vi "Measure-Scope.vi"(0 "VISA resource name":refnum<visa-resource-name>, 1 "Avg Num Samples":dbl, 3 "Boolean":bool, 5 "Channel1 (0:Channel1)":u16(ring) items=["Channel1", "Channel2", "Channel3", "Channel4", "Math1", "Math2", "Math3", "Math3", "Reference1", "Reference2", "Reference3", "Reference4"], 9 "Gate Index":i32, 11 "Gate Length":i32=1000, 12 "error in (no error)":errorcluster) -> (4 "Full Waveform":waveform(dbl)(graph)={"t0"=timestamp(1.815305999999491e-07 s since 1904-01-01), "dt"=5e-07, "Y"=array[10000 elements]}, 6 "Gate":dbl[](graph), 8 "Signal Duration (ns)":dbl, 10 "Signal Arrival (ns)":dbl, 14 "Sum of Intensity (V)":dbl, 15 "Wait Time (ms)":dbl)   [LabVIEW 2018]
uses:
  <instrlib>/Tektronix 7000 Series/Public/Data/Read Waveform Measurement (More).vi
  <instrlib>/Tektronix 7000 Series/Public/Data/Read (Single Waveform).vi
  <instrlib>/Tektronix 7000 Series/Tektronix 7000 Series.lvlib
panel:
  out "Area (V*s)":dbl
  in  "Function(0:Amplitude)":u16(ring) items=["Area", "Burst Width", "Cyc Area", "Phase"]
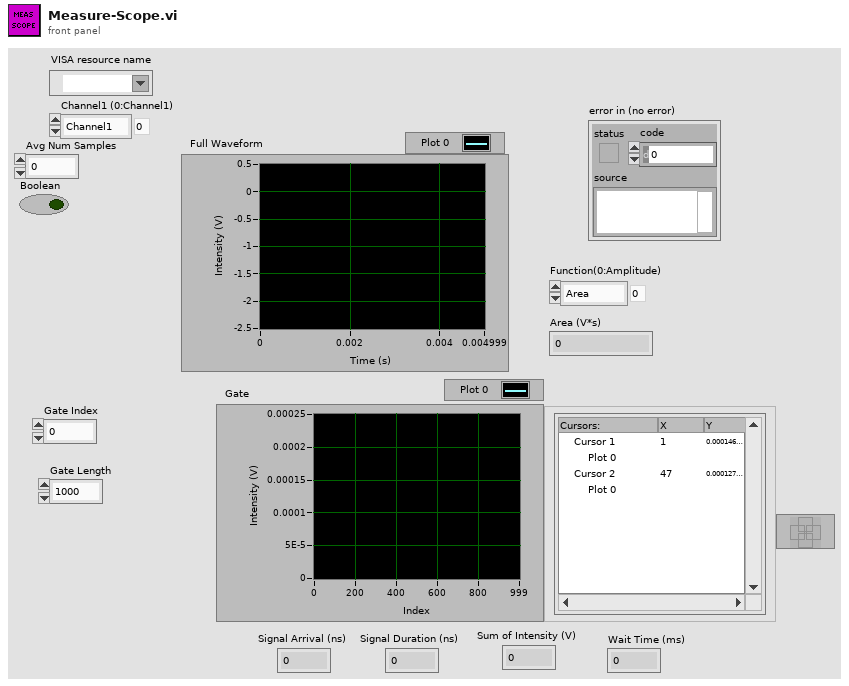
[diagram p1: front panel]
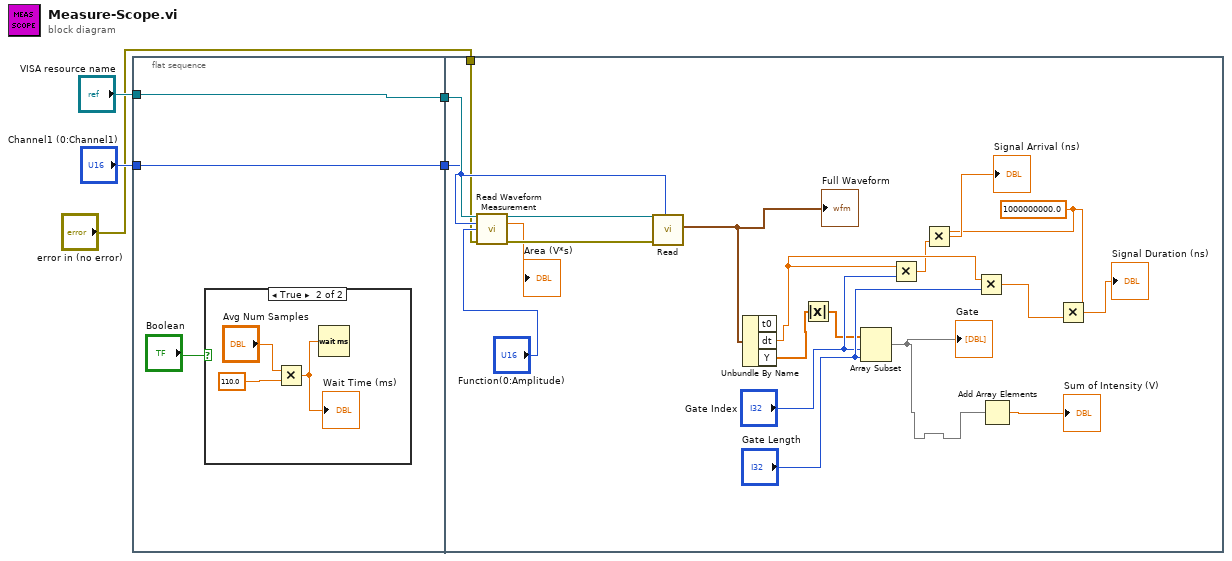
[diagram p0: block diagram]
diagram:
  n1 = flat-sequence {
    tunnel: "VISA resource name" -> [w8]
    tunnel: "Channel1 (0:Channel1)" -> [w7]
    tunnel: [w8] -> w3
    tunnel: [w7] -> w2
    tunnel: w3 -> [w18]
    tunnel: w2 -> [w17]
    tunnel: "error in (no error)" -> [w15]
    frame #0 {
      n2 = case shown="True" "Boolean" {
        frame False {
        }
        frame True {
          n3 = Multiply(x="Avg Num Samples", y=110.0) -> (x*y=w11:dbl)
          "Wait Time (ms)" <- w11
          n4 = Wait (ms)(milliseconds to wait=w11) -> ()  [unwired: 1 out]
        }
      }
    }
    frame #1 {
      w19 = 1000000000.0 ("x")
      n5 = call-poly <instrlib>:"Read Waveform Measurement.vi"("VISA resource name"=w18, "Channel1 (0:Channel1)"=w17, "Function(0:Amplitude)"="Function(0:Amplitude)", "error in (no error)"=w15) -> ("VISA resource name out"=w22:refnum<visa-resource-name>, "Measurement"=→"Area (V*s)":dbl, "error out"=w21:errorcluster)  [unwired: 9 in]
      n6 = call-poly <instrlib>:"Read.vi"("error in (no error)"=w21, "Channel (0: Channel 1)"=w17, "VISA resource name"=w22) -> ("Waveform Data"=w24:waveform(dbl))  [unwired: 6 in, 2 out]
      "Full Waveform" <- w24
      n7 = Unbundle By Name(w24) -> ("dt"=w30:dbl, "Y"=w13:dbl[])  [unwired: 1 out]
      n8 = Absolute Value(x=w13) -> (abs(x)=w12:dbl[])
      n9 = Array Subset(array=w12, index="Gate Index", length="Gate Length") -> (w14:dbl[])
      "Gate" <- w14
      n10 = Multiply(x=w30, y="Gate Index") -> (x*y=w28:dbl)
      n11 = Multiply(x=w19, y=w28) -> (x*y=→"Signal Arrival (ns)":dbl)
      n12 = Multiply(x=w30, y="Gate Length") -> (x*y=w31:dbl)
      n13 = Add Array Elements(numeric array=w14) -> (sum=→"Sum of Intensity (V)":dbl)
      n14 = Multiply(x=w19, y=w31) -> (x*y=→"Signal Duration (ns)":dbl)
    }
  }
